vi "旧坐标转换为新坐标.vi"(1 "新坐标":cluster{"X":dbl, "Y":dbl}) -> (0 "新坐标":cluster{"X":dbl, "Y":dbl} {"Y" format="%#_6f"})   [LabVIEW 2014]
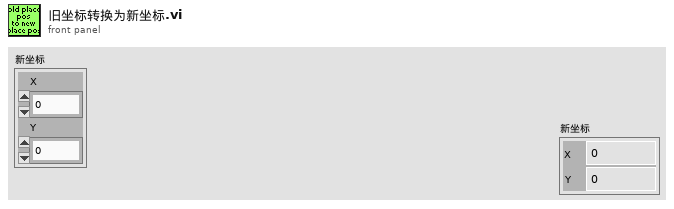
[diagram p1: front panel]
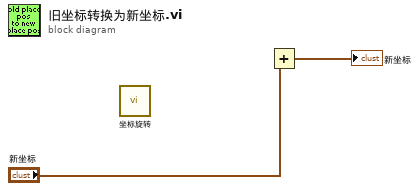
[diagram p0: block diagram]
diagram:
  n1 = call "坐标旋转.vi"() -> ()  [unwired: 11 in, 1 out]
  n2 = Add(y="新坐标") -> (x+y=→"新坐标":cluster{"X":dbl, "Y":dbl})  [unwired: 1 in]
